vi "Read 2D Compass Property Array.vi"(8 "error in (no error)":errorcluster, 11 "2D Compass.lvclass in":refnum<class "2D Compass.lvclass">) -> (0 "error out":errorcluster, 2 "2D Compass Array":T1, 3 "2D Compass.lvclass out":refnum<class "2D Compass.lvclass">)   [LabVIEW 2020, in "2D Compass.lvclass"]
uses:
  <vilib>/Math Plots/2D Math Plots/2D Compass/2D Compass/2D Compass.lvclass
  <vilib>/Math Plots/2D Math Plots/2D Compass/2D Compass/Typedef/2D Compass Property Array.ctl
  <vilib>/Math Plots/2D Math Plots/2D Compass/2D Compass/Typedef/2D Compass Property.ctl
  <vilib>/Math Plots/2D Math Plots/2D Compass/2D Compass/2D Compass.lvclass/2D Compass.ctl
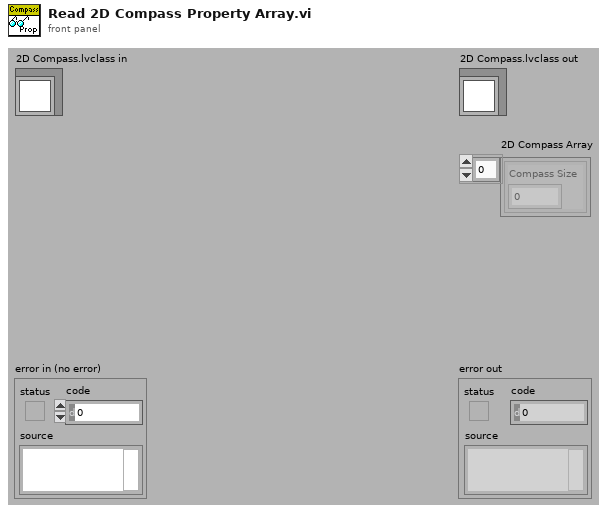
[diagram p1: front panel]
types:
  T1 = typedef "2D Compass.lvclass/2D Compass Property Array.ctl" = T2[]
  T2 = typedef "2D Compass.lvclass/2D Compass Property.ctl" = cluster{"Compass Size":dbl}
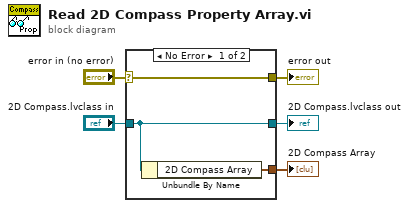
[diagram p0: block diagram]
diagram:
  n1 = case shown="No Error" "error in (no error)" {
    selector: "error in (no error)" -> [w8 w9]
    tunnel: [w8 w9] -> w4
    tunnel: [w7 w10] -> w2
    tunnel: "2D Compass.lvclass in" -> [w7 w10]
    tunnel: [w6 _] -> w1
    frame No Error {
      n2 = Unbundle By Name(w7) -> ("2D Compass Array"=w6:T1)
    }
    frame Error {
    }
  }
  "error out" <- w4
  "2D Compass.lvclass out" <- w2
  "2D Compass Array" <- w1
